vi "Configure Test Runner.vi"(8 "error in (no error)":errorcluster, 10 "Run Tests In Parallel?":bool, 11 "Execution API In":refnum<class "Execution API.lvclass">) -> (0 "error out":errorcluster, 3 "Execution API Out":refnum<class "Execution API.lvclass">)   [LabVIEW 2020, in "Execution API.lvclass"]
doc: "Configure the number of test runners to launch in parallel. The configuration must be made before running the tests."
uses:
  Execution API.lvclass
  Execution API.lvclass/Execution API.ctl
  Parallel Test Runner/Parallel Test Runner.lvclass
  C:/git/astemes-lunit/source/Framework/Test Runner/Test Runner.lvclass
  Single Thread Test Runner/Single Thread Test Runner.lvclass
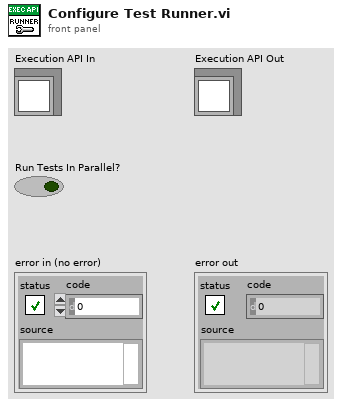
[diagram p1: front panel]
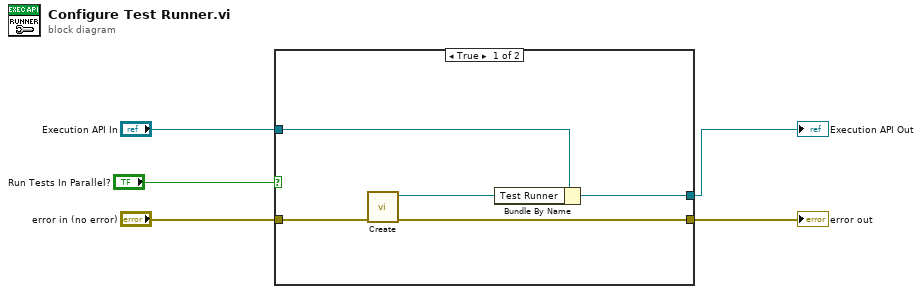
[diagram p0: block diagram]
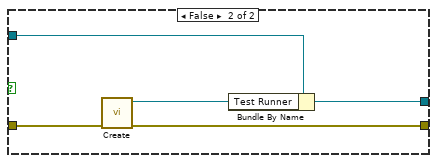
[diagram p2: hidden frame]
diagram:
  n1 = case shown="True" "Run Tests In Parallel?" {
    tunnel: "Execution API In" -> [w7 w12]
    tunnel: "error in (no error)" -> [w10 w15]
    tunnel: [w6 w11] -> w3
    tunnel: [w9 w14] -> w1
    frame True {
      n2 = call "Create.vi"("error in (no error)"=w10) -> ("error out"=w6:errorcluster, "Parallell Test Runner out"=w8:refnum<class "Parallel Test Runner.lvclass">)  [unwired: 9 in]
      n3 = Bundle By Name(cluster=w7, "Test Runner"=w8) -> (w9:refnum<class "Execution API.lvclass">)
    }
    frame False {
      n4 = call "Create.vi"("error in (no error)"=w15) -> ("error out"=w11:errorcluster, "Single Thread Test Runner out"=w13:refnum<class "Single Thread Test Runner.lvclass">)  [unwired: 9 in]
      n5 = Bundle By Name(cluster=w12, "Test Runner"=w13) -> (w14:refnum<class "Execution API.lvclass">)
    }
  }
  "error out" <- w3
  "Execution API Out" <- w1
